vi "Get Test Sequence.vi"(8 "error in (no error)":errorcluster caption="entrée d'erreur (pas d'erreur)", 11 "Sequencer (Default) en entrée":refnum<class "Sequencer (Default).lvclass">) -> (0 "error out":errorcluster caption="sortie d'erreur", 2 "Test Sequence":T1(array[cluster]), 3 "Sequencer (Default) en sortie":refnum<class "Sequencer (Default).lvclass">)   [LabVIEW 2020, in "Library Core.lvlib" / "Sequencer (Default).lvclass"]
uses:
  Sequencer (Default).lvclass
  Sequencer (Default).lvclass/Sequencer (Default).ctl
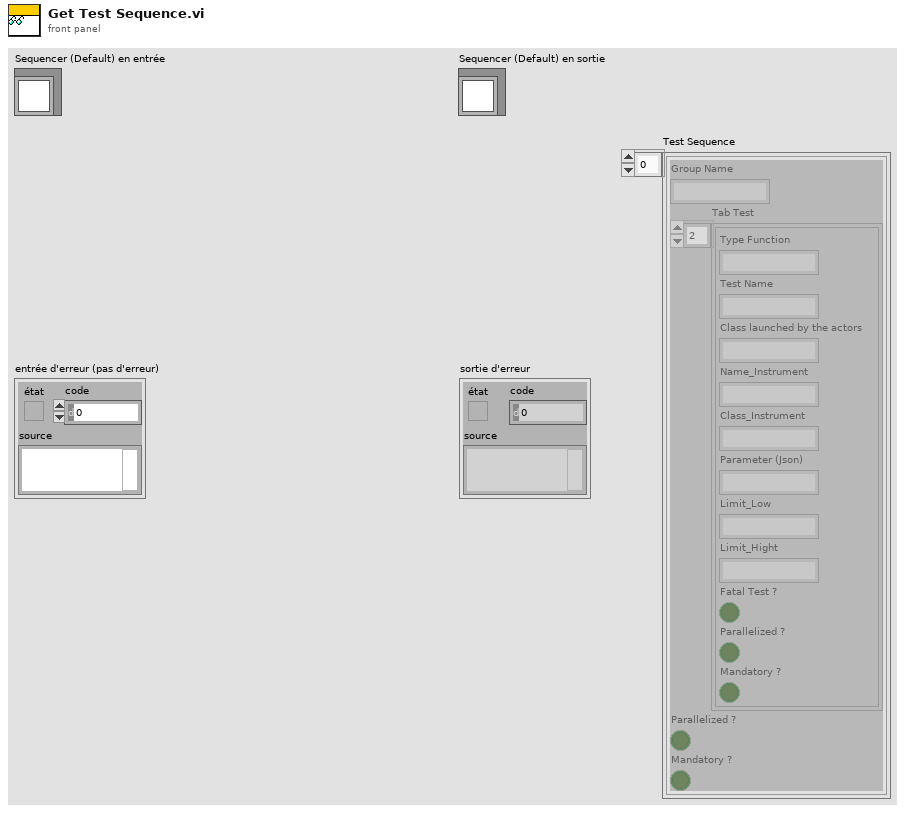
[diagram p1: front panel]
types:
  T1 = cluster{"Group Name":string, "Tab Test":cluster{"Type Function":string, "Test Name":string, "Class launched by the actors ":string, "Name_Instrument":string, "Class_Instrument":string, "Parameter (Json)":string, "Limit_Low":string, "Limit_Hight":string, "Fatal Test ?":bool, "Parallelized ?":bool, "Mandatory ?":bool}[], "Parallelized ?":bool, "Mandatory ?":bool}[]
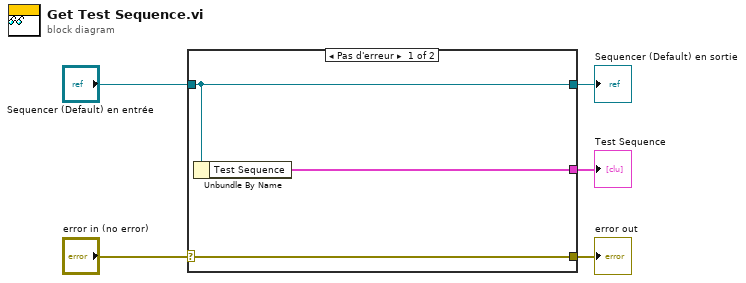
[diagram p0: block diagram]
diagram:
  n1 = case shown="Pas d'erreur" "error in (no error)" {
    selector: "error in (no error)" -> [w8 w9]
    tunnel: [w8 w9] -> w4
    tunnel: [w7 w10] -> w2
    tunnel: "Sequencer (Default) en entrée" -> [w7 w10]
    tunnel: [w6 _] -> w1
    frame No Error {
      n2 = Unbundle By Name(w7) -> ("Test Sequence"=w6:T1)
    }
    frame Error {
    }
  }
  "error out" <- w4
  "Sequencer (Default) en sortie" <- w2
  "Test Sequence" <- w1
